vi "Initial Orientation.vi"(1 "data AGM - XYZ":dbl[](array[numeric])) -> (0 "Quaternion":dbl[](array[numeric]))   [LabVIEW 2021, in "IMU Processing.lvlib"]
uses:
  IMU Processing.lvlib
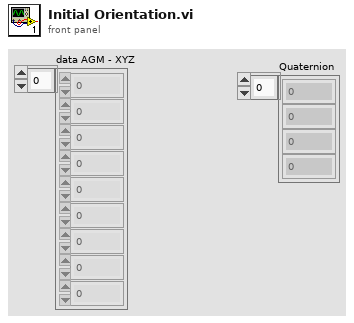
[diagram p1: front panel]
types:
  T1 = typedef "NI_Matrix.lvlib/RealMatrix.ctl" = dbl[][]
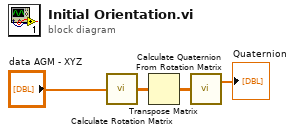
[diagram p0: block diagram]
diagram:
  n1 = call "Calculate Rotation Matrix.vi"("data AGM - XYZ"="data AGM - XYZ") -> ("Rotation Matrix"=w3:T1)
  n2 = Transpose Matrix(1:w3) -> (0:w2:T1)
  n3 = call "Calculate Quaternion From Rotation Matrix.vi"("Rotation Matrix"=w2) -> ("Quaternion"=→"Quaternion":dbl[])  [unwired: 1 out]
